vi "Play_Audio.vi"(8 "error in (no error)":errorcluster, 10 "Parameters":string, 11 "reference in":refnum<class "Test_Flux_Capacitor.lvclass">) -> (0 "error out":errorcluster, 2 "Result":dbl, 3 "reference out":refnum<class "Test_Flux_Capacitor.lvclass">)   [LabVIEW 2022 SP3, in "Test_Flux_Capacitor.lvlib" / "Test_Flux_Capacitor.lvclass"]
uses:
  Test_Flux_Capacitor.lvclass
  ParameterTypes/PlayTone.ctl
  ParameterTypes/DMM_ACV.ctl
  Components/SwitchBase.lvlibp/SwitchBase.lvclass
  Components/DMM_Keysight_34980A.lvlibp/DMM_Keysight_34980A.lvclass
  <vilib>/JDP Science/JSONtext/JSONtext.lvlib
panel:
  in  "Parameter_Type":T1={"Pre_Switch"="", "Post_Switch"="", "Wait (msec)"=0, "Scale"=0.0, "DMM_ACV"={"Range"=enum."Auto", "Bandwidth"=enum."3 Hz", "Samples"=1, "dt (s)"=0.0, "Timeout (s)"=10000.0}, "Volume"=0, "Tone"=enum."High"}
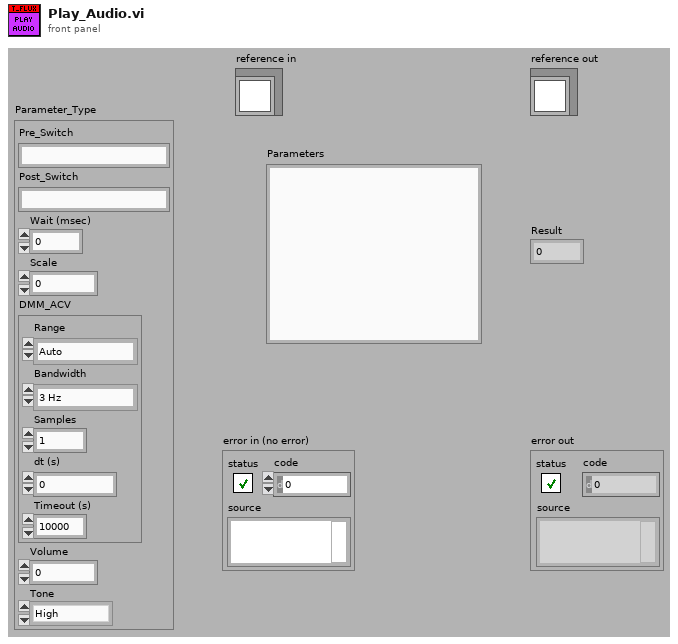
[diagram p1: front panel]
types:
  T1 = typedef "Test_Flux_Capacitor.lvlib/Test_Flux_Capacitor.lvclass/PlayTone.ctl" = cluster{"Pre_Switch":string, "Post_Switch":string, "Wait (msec)":u32, "Scale":dbl, "DMM_ACV":T2, "Volume":u8, "Tone":enum16{"High", "Low"}}
  T2 = typedef "Test_Flux_Capacitor.lvlib/Test_Flux_Capacitor.lvclass/DMM_ACV.ctl" = cluster{"Range":enum16{"100 mV", "1 V", "10 V", "100 V", "300 V", "Auto", "Minimum", "Maximum", "Default"}, "Bandwidth":enum16{"3 Hz", "20 Hz", "200 Hz", "Minimum", "Maximum"}, "Samples":u32, "dt (s)":dbl, "Timeout (s)":dbl}
  T3 = typedef "Test_Flux_Capacitor.lvlib/Test_Flux_Capacitor.lvclass/ObjectAttributes.ctl" = cluster{"Config":T4, "DMM":refnum<class "DMM_Keysight_34980A.lvclass">, "LCR":refnum<class "LCR_BK891.lvclass">, "PSU":refnum<class "PSU_Base.lvclass">, "Switch_Manager":refnum<class "SwitchBase.lvclass">, "FRAM":string, "Flux_Capacitor":refnum<class "Flux_Capacitor.lvclass">, "Frequency_Counter":refnum<class "Frequency_Counter_Base.lvclass">, "JTAG":refnum<class "JTAG_Base.lvclass">}
  T4 = typedef "Test_Flux_Capacitor.lvlib/Test_Flux_Capacitor.lvclass/Config.ctl" = cluster{"default":string}
  T5 = enum16{"100 mV", "1 V", "10 V", "100 V", "300 V", "Auto", "Minimum", "Maximum", "Default"}
  T6 = enum16{"3 Hz", "20 Hz", "200 Hz", "Minimum", "Maximum"}
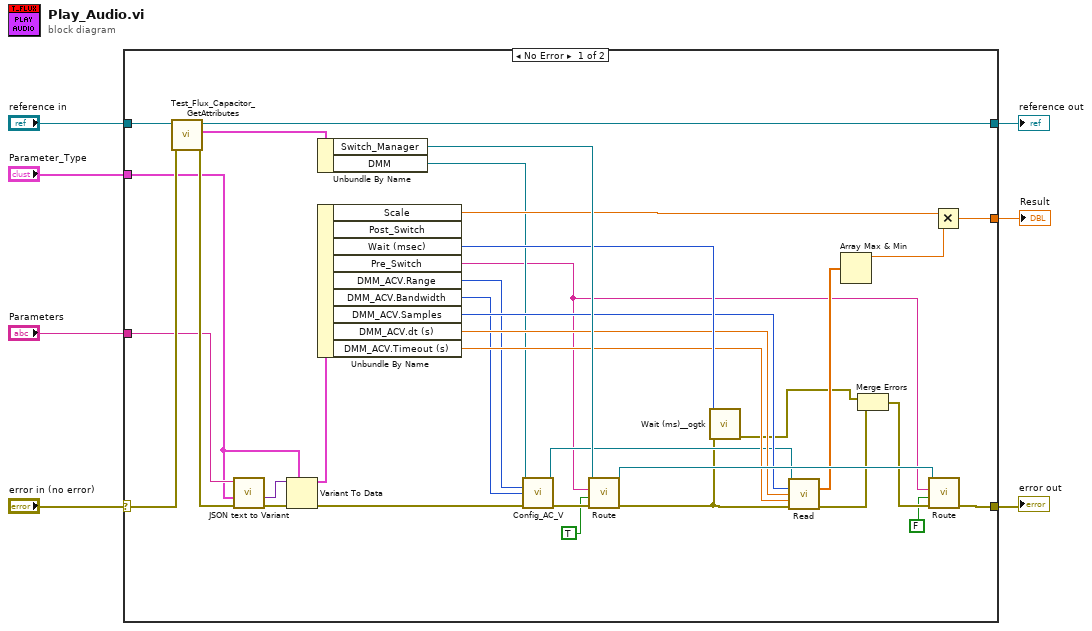
[diagram p0: block diagram]
diagram:
  n1 = case shown="No Error" "error in (no error)" {
    selector: "error in (no error)" -> [w41 w43]
    tunnel: [w31 w43] -> w6
    tunnel: [w39 w42] -> w4
    tunnel: "reference in" -> [w40 w42]
    tunnel: "Parameters" -> [w15 _]
    tunnel: "Parameter_Type" -> [w14 _]
    tunnel: [w32 _] -> w1
    frame No Error {
      n2 = call "Test_Flux_Capacitor_GetAttributes.vi"("error in (no error)"=w41, "reference in"=w40) -> ("error out"=w17:errorcluster, "Data"=w38:T3, "reference out"=w39:refnum<class "Test_Flux_Capacitor.lvclass">)  [unwired: 6 in, 1 out]
      n3 = call <vilib>:"JSON text to Variant.vi"("error in (no error)"=w17, "Data Type"=w14, "JSON"=w15) -> ("error out"=w16:errorcluster, "Variant out"=w13:variant)  [unwired: 7 in]
      n4 = Variant To Data(error in=w16, type=w14, Variant=w13) -> (data=w37:T1, error out=w27:errorcluster)
      n5 = Unbundle By Name(w38) -> ("Switch_Manager"=w36:refnum<class "SwitchBase.lvclass">, "DMM"=w25:refnum<class "DMM_Keysight_34980A.lvclass">)
      n6 = Unbundle By Name(w37) -> ("Scale"=w33:dbl, "Wait (msec)"=w35:u32, "Pre_Switch"=w12:string, "DMM_ACV.Range"=w23:T5, "DMM_ACV.Bandwidth"=w22:T6, "DMM_ACV.Samples"=w30:u32, "DMM_ACV.dt (s)"=w29:dbl, "DMM_ACV.Timeout (s)"=w28:dbl)  [unwired: 1 out]
      n7 = call-dynamic "Config_AC_V.vi"("reference in"=w25, "Range (5:Auto)"=w23, "Bandwidth (1:20 Hz)"=w22, "error in (no error)"=w27) -> ("reference in"=w24:refnum<class "DMM_Keysight_34980A.lvclass">, "error out"=w26:errorcluster)  [unwired: 10 in]
      n8 = call-dynamic "Route.vi"("error in (no error)"=w26, "Connect"=TRUE, "channel 1"=w12, "reference in"=w36) -> ("error out"=w8:errorcluster, "reference in"=w34:refnum<class "SwitchBase.lvclass">)  [unwired: 6 in]
      n9 = call <userlib>:"Wait (ms)__ogtk.vi"("error in (no error)"=w8, "milliseconds to wait"=w35) -> ("error out"=w9:errorcluster)  [unwired: 8 in, 1 out]
      n10 = call-dynamic "Read.vi"("reference in"=w24, "Samples"=w30, "dt"=w29, "Timeout (10 s)"=w28, "error in (no error)"=w8) -> ("Measurement"=w19:dbl[], "error out"=w21:errorcluster)  [unwired: 7 in, 2 out]
      n11 = Array Max & Min(array=w19) -> (max value=w18:dbl)  [unwired: 3 out]
      n12 = Merge Errors(w9, w21) -> (w20:errorcluster)
      n13 = call-dynamic "Route.vi"("error in (no error)"=w20, "Connect"=FALSE, "channel 1"=w12, "reference in"=w34) -> ("error out"=w31:errorcluster)  [unwired: 6 in, 1 out]
      n14 = Multiply(x=w33, y=w18) -> (x*y=w32:dbl)
    }
    frame Error {
    }
  }
  "Result" <- w1
  "error out" <- w6
  "reference out" <- w4
